vi "Time averaged data pairs.vi"(3 "Averaging period (ms)":dbl=100.0, 4 "Time Cluster 2":T1, 5 "Time Cluster 1":T1) -> (0 "Centre Time (s)":dbl[](array[numeric]), 1 "Eng Values 2":dbl[](array[numeric]), 2 "Eng Values 1":dbl[](array[numeric]))   [LabVIEW 2022 SP3]
uses:
  Controls/Time_Trace_Cluster.ctl
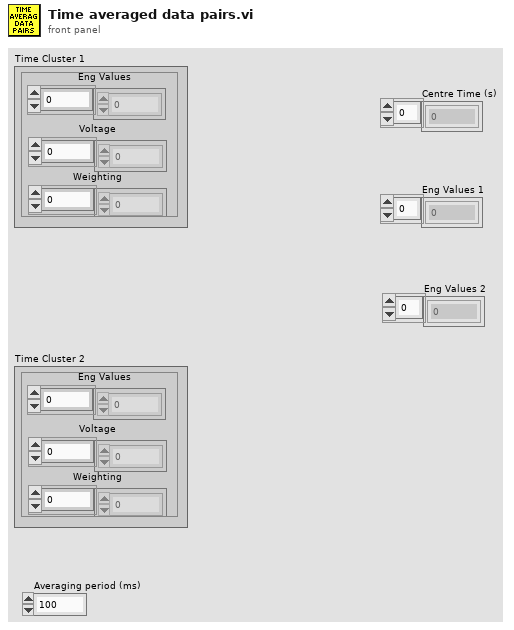
[diagram p1: front panel]
types:
  T1 = typedef "Time_Trace_Cluster.ctl" = cluster{"Weighting":dbl[], "Voltage":dbl[], "Eng Values":dbl[]}
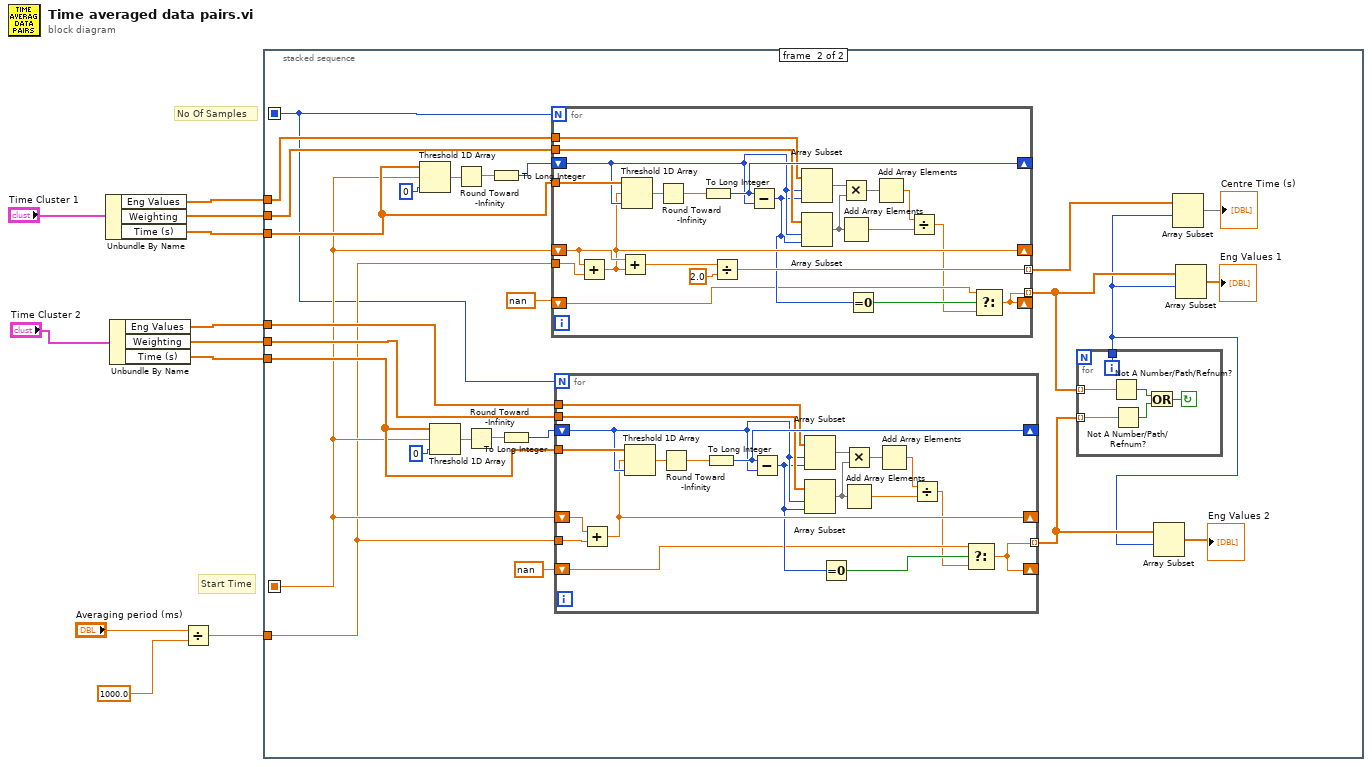
[diagram p0: block diagram]
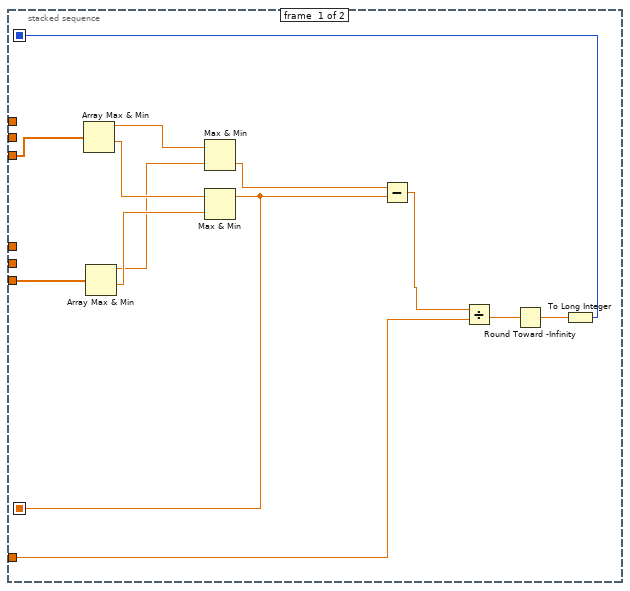
[diagram p2: hidden frame]
diagram:
  # "No Of Samples"
  # "Start Time"
  n1 = Unbundle By Name("Time Cluster 1") -> ("Eng Values"=w4:dbl[], "Weighting"=w9:dbl[], "Time (s)"=w3:dbl[])
  n2 = Unbundle By Name("Time Cluster 2") -> ("Eng Values"=w2:dbl[], "Weighting"=w1:dbl[], "Time (s)"=w8:dbl[])
  n3 = Divide(x="Averaging period (ms)", y=1000.0) -> (x/y=w5:dbl)
  n4 = stacked-sequence {
    seq-local: [w14 _] -> [_ w36]
    seq-local: [w13 _] -> [_ w34]
    tunnel: w9 -> [_ w45]
    tunnel: w8 -> [w24 w38]
    tunnel: w5 -> [w17 w35]
    tunnel: w4 -> [_ w46]
    tunnel: w3 -> [w12 w44]
    tunnel: w2 -> [_ w43]
    tunnel: w1 -> [_ w42]
    frame #0 {
      n5 = Array Max & Min(array=w12) -> (max value=w21:dbl, min value=w23:dbl)  [unwired: 2 out]
      n6 = Array Max & Min(array=w24) -> (max value=w20:dbl, min value=w22:dbl)  [unwired: 2 out]
      n7 = Max & Min(x=w21, y=w20) -> (min(x,y)=w19:dbl)  [unwired: 1 out]
      n8 = Max & Min(x=w23, y=w22) -> (max(x,y)=w14:dbl)  [unwired: 1 out]
      n9 = Subtract(x=w19, y=w14) -> (x-y=w18:dbl)
      n10 = Divide(x=w18, y=w17) -> (x/y=w16:dbl)
      n11 = Round Toward -Infinity(1:w16) -> (0:w15:dbl)
      n12 = To Long Integer(number=w15) -> (32bit integer=w13:i32)
    }
    frame #1 {
      n13 = Threshold 1D Array(1:0 ("start index (0)"), 2:w36, 3:w44) -> (0:w48:dbl)
      n14 = Threshold 1D Array(1:0 ("start index (0)"), 2:w36, 3:w38) -> (0:w41:dbl)
      n15 = Round Toward -Infinity(1:w48) -> (0:w49:dbl)
      n16 = Round Toward -Infinity(1:w41) -> (0:w40:dbl)
      n17 = To Long Integer(number=w49) -> (32bit integer=w47:i32)
      n18 = To Long Integer(number=w40) -> (32bit integer=w37:i32)
      n19 = for {
        N: w34 -> [_]
        tunnel: w35 -> [w99]
        shift-right: [w85] -> _
        shift-left: w36 -> [w86]
        tunnel: w44 -> [w98]
        shift-right: [w95] -> _
        shift-left: w47 -> [w92]
        tunnel: w46 -> [w94]
        tunnel: w45 -> [w93]
        tunnel: [w82] -> w31 mode=indexing
        shift-right: [w77] -> _
        shift-left: nan -> [w79]
        tunnel: [w77] -> w29 mode=indexing
        n20 = Add(x=w86, y=w99) -> (x+y=w85:dbl)
        n21 = Add(x=w86, y=w85) -> (x+y=w84:dbl)
        n22 = Threshold 1D Array(1:w92, 2:w85, 3:w98) -> (0:w97:dbl)
        n23 = Round Toward -Infinity(1:w97) -> (0:w96:dbl)
        n24 = To Long Integer(number=w96) -> (32bit integer=w95:i32)
        n25 = Divide(x=w84, y=2.0) -> (x/y=w82:dbl)
        n26 = Subtract(x=w95, y=w92) -> (x-y=w80:i32)
        n27 = Array Subset(array=w94, index=w92, length=w80) -> (w91:dbl[])
        n28 = Array Subset(array=w93, index=w92, length=w80) -> (w89:dbl[])
        n29 = Multiply(x=w91, y=w89) -> (x*y=w90:dbl[])
        n30 = Add Array Elements(numeric array=w89) -> (sum=w88:dbl)
        n31 = Equal To 0?(x=w80) -> (x = 0?=w81:bool)
        n32 = Add Array Elements(numeric array=w90) -> (sum=w87:dbl)
        n33 = Divide(x=w87, y=w88) -> (x/y=w78:dbl)
        n34 = Select(t=w79, s=w81, f=w78) -> (s? t:f=w77:dbl)
      }
      n35 = for {
        N: w34 -> [_]
        shift-right: [w63] -> _
        shift-left: w36 -> [w64]
        tunnel: w38 -> [w76]
        shift-right: [w73] -> _
        shift-left: w37 -> [w70]
        tunnel: w43 -> [w72]
        tunnel: w42 -> [w71]
        tunnel: w35 -> [w62]
        shift-right: [w57] -> _
        shift-left: nan -> [w59]
        tunnel: [w57] -> w27 mode=indexing
        n36 = Add(x=w64, y=w62) -> (x+y=w63:dbl)
        n37 = Threshold 1D Array(1:w70, 2:w63, 3:w76) -> (0:w75:dbl)
        n38 = Round Toward -Infinity(1:w75) -> (0:w74:dbl)
        n39 = To Long Integer(number=w74) -> (32bit integer=w73:i32)
        n40 = Subtract(x=w73, y=w70) -> (x-y=w61:i32)
        n41 = Array Subset(array=w72, index=w70, length=w61) -> (w69:dbl[])
        n42 = Array Subset(array=w71, index=w70, length=w61) -> (w67:dbl[])
        n43 = Equal To 0?(x=w61) -> (x = 0?=w60:bool)
        n44 = Multiply(x=w69, y=w67) -> (x*y=w68:dbl[])
        n45 = Add Array Elements(numeric array=w67) -> (sum=w66:dbl)
        n46 = Add Array Elements(numeric array=w68) -> (sum=w65:dbl)
        n47 = Divide(x=w65, y=w66) -> (x/y=w58:dbl)
        n48 = Select(t=w59, s=w60, f=w58) -> (s? t:f=w57:dbl)
      }
      n49 = for {
        tunnel: w29 -> [w56] mode=indexing
        tunnel: w27 -> [w55] mode=indexing
        tunnel: [w51] -> w25
        i -> [w51]
        stop <- w52 continue-if-true
        n50 = Not A Number/Path/Refnum?(number/path/refnum=w56) -> (NaN/Path/Refnum?=w53:bool)
        n51 = Not A Number/Path/Refnum?(number/path/refnum=w55) -> (NaN/Path/Refnum?=w54:bool)
        n52 = Or(x=w53, y=w54) -> (x .or. y?=w52:bool)
      }
      n53 = Array Subset(array=w27, index=w25) -> (→"Eng Values 2":dbl[])  [unwired: 1 in]
      n54 = Array Subset(array=w31, index=w25) -> (→"Centre Time (s)":dbl[])  [unwired: 1 in]
      n55 = Array Subset(array=w29, index=w25) -> (→"Eng Values 1":dbl[])  [unwired: 1 in]
    }
  }
